vi "DataFlowAverage.vi"(9 "timer":u32, 10 "name":string, 11 "data in":variant) -> (2 "average":dbl, 3 "data out":variant)   [LabVIEW 2017, in "Benchmarking.lvlib"]
uses:
  <vilib>/addons/InsightCM/Devices/Shared/Common/Benchmarking/Benchmarking.lvlib
  <vilib>/addons/PointValueMap/subVIs/Point_Write_double.vi
  <vilib>/addons/PointValueMap/PointValueMap.lvlib
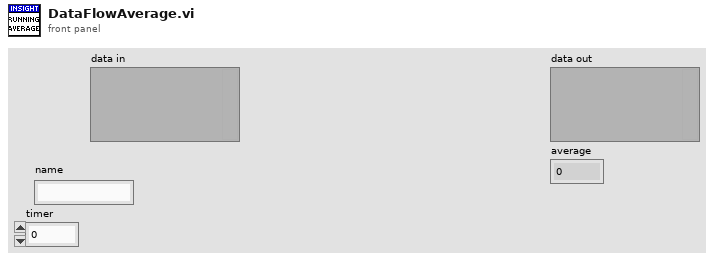
[diagram p1: front panel]
types:
  T1 = typedef "PointValueMap.lvlib/PointMap.ctl" = refnum<data-value>
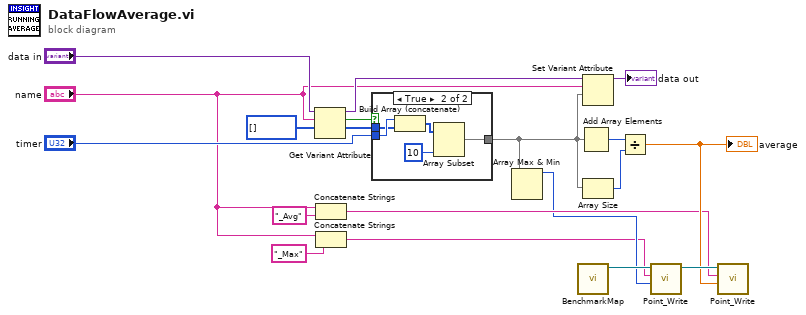
[diagram p0: block diagram]
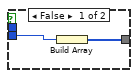
[diagram p2: hidden frame]
diagram:
  n1 = Get Variant Attribute(Variant="data in", name="name", default value (empty Variant)=u32[] []) -> (duplicate Variant=w15:variant, found=w7:bool, value=w16:u32[])  [unwired: 1 in, 1 out]
  n2 = Concatenate Strings("name", "_Avg" ("string")) -> (w3:string)
  n3 = Concatenate Strings("name", "_Max" ("string")) -> (w1:string)
  n4 = case shown="True" w7 {
    tunnel: w16 -> [_ w22]
    tunnel: "timer" -> [w21 w23]
    tunnel: [w20 w24] -> w8
    frame False {
      n5 = Build Array(w21) -> (w20:u32[])
    }
    frame True {
      n6 = Build Array (concatenate)(w23, w22) -> (w25:u32[])
      n7 = Array Subset(array=w25, length=10) -> (w24:u32[])  [unwired: 1 in]
    }
  }
  n8 = Array Max & Min(array=w8) -> (max value=w2:u32)  [unwired: 3 out]
  n9 = call <vilib>:"BenchmarkMap.vi"() -> ("benchmark map"=w6:T1)  [unwired: 10 in, 1 out]
  n10 = Add Array Elements(numeric array=w8) -> (sum=w14:u32)
  n11 = Set Variant Attribute(Variant=w15, name="name", value=w8) -> (Variant out=→"data out":variant)  [unwired: 1 in, 2 out]
  n12 = Array Size(array=w8) -> (size(s)=w13:i32)
  n13 = Divide(x=w14, y=w13) -> (x/y=w4:dbl)
  "average" <- w4
  n14 = call-poly <vilib>:"Point_Write.vi"("Value"=w2, "Tag"=w1, "Map"=w6) -> ("Map Out"=w5:T1)  [unwired: 7 in, 1 out]
  n15 = call-poly <vilib>:"Point_Write.vi"("Value"=w4, "Tag"=w3, "Map"=w5) -> ()  [unwired: 7 in, 2 out]
